vi "Get Video Image.vi"(8 "error in (no error)":errorcluster, 9 "Wait For Next Image?":bool=TRUE, 10 "Flip Image?":bool=TRUE, 11 "queue in":refnum<queue>) -> (0 "error out":errorcluster, 1 "Image Is New?":bool, 2 "Video Image Pixels (U32)":u32[][](array[numeric]), 3 "Video Image":T1(plugin-control))   [LabVIEW 2010, in "Kinect_API.lvlib"]
uses:
  Kinect_API.lvlib
  <vilib>/vision/Image Controls.llb/IMAQ Image.ctl
  <vilib>/vision/NI_Vision_Development_Module.lvlib
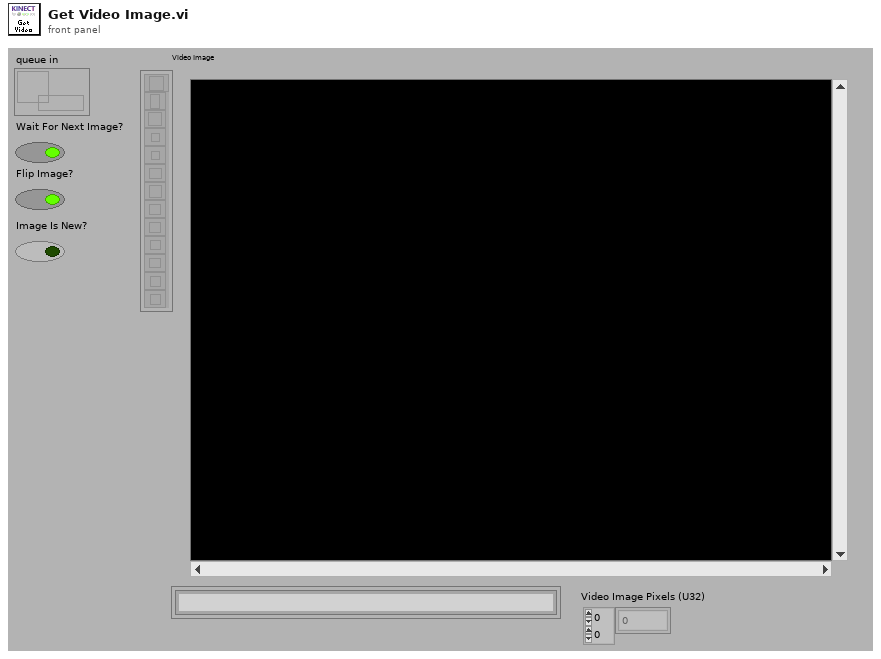
[diagram p1: front panel]
types:
  T1 = typedef "IMAQ Image.ctl" = refnum<image>
  T2 = typedef "Image Type" = u32
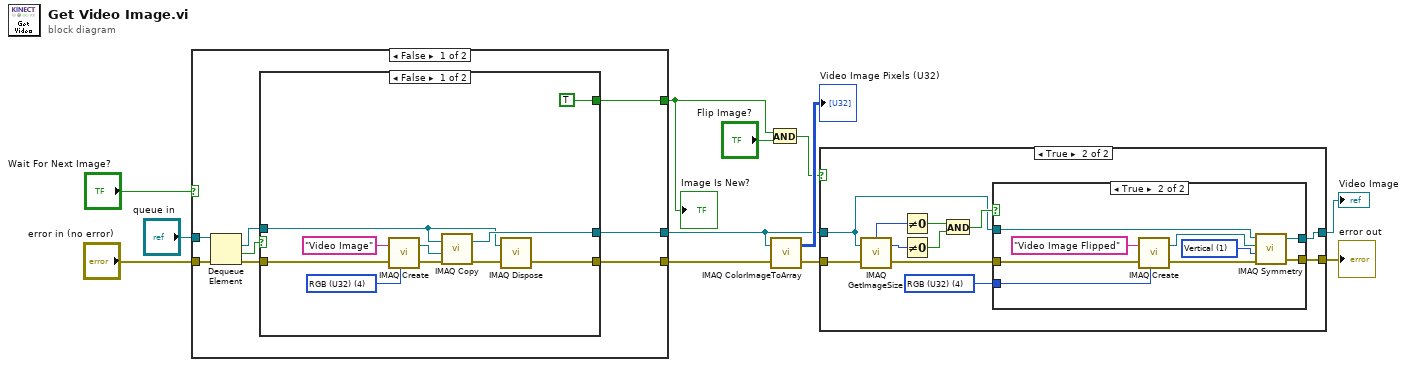
[diagram p0: block diagram]
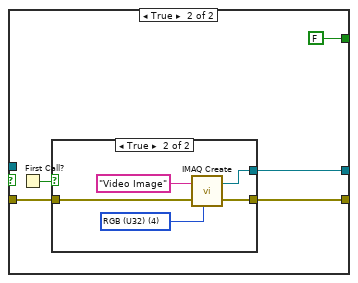
[diagram p4: hidden frame]
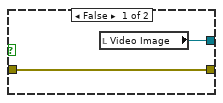
[diagram p5: hidden frame]
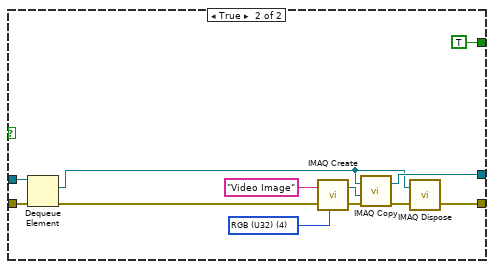
[diagram p6: hidden frame]
diagram:
  n1 = case shown="False" "Wait For Next Image?" {
    tunnel: "error in (no error)" -> [w16 w54]
    tunnel: [w18 w48] -> w7
    tunnel: [w19 w44] -> w8
    tunnel: [w20 TRUE] -> w2
    tunnel: "queue in" -> [w17 w52]
    frame False {
      n2 = Dequeue Element(queue=w17, error in (no error)=w16) -> (element=w13:T1, timed out?=w14:bool, error out=w15:errorcluster)  [unwired: 1 in, 1 out]
      n3 = case shown="False" w14 {
        tunnel: [w24 w31] -> w18
        tunnel: w15 -> [w21 w33]
        tunnel: [w23 w32] -> w19
        tunnel: [TRUE FALSE] -> w20
        tunnel: w13 -> [w22 _]
        frame False {
          w26 = T2 4 items=["Grayscale (U8)", "Grayscale (I16)", "Grayscale (SGL)", "Complex (CSG)", "RGB (U32)", "HSL (U32)", "RGB (U64)", "Grayscale (U16)"] ("Image Type")
          n4 = call "IMAQ Create"("Image Name"="Video Image", "Image Type"=w26, "error in (no error)"=w21) -> ("New Image"=w28:T1, "error out"=w27:errorcluster)  [unwired: 2 in]
          n5 = call "IMAQ Copy"("error in (no error)"=w27, "Image Dst"=w28, "Image Src"=w22) -> ("error out"=w25:errorcluster, "Image Dst Out"=w24:T1)  [unwired: 3 in]
          n6 = call "IMAQ Dispose"("Image"=w22, "error in (no error)"=w25) -> ("error out"=w23:errorcluster)  [unwired: 4 in]
        }
        frame True {
          n7 = First Call?() -> (First Call?: T/F=w34:bool)
          n8 = case shown="True" w34 {
            tunnel: [w37 w38] -> w31
            tunnel: w33 -> [w36 w40]
            tunnel: [w36 w39] -> w32
            frame False {
              n9 = local read "Video Image"() -> (w37:T1)
            }
            frame True {
              w41 = T2 4 items=["Grayscale (U8)", "Grayscale (I16)", "Grayscale (SGL)", "Complex (CSG)", "RGB (U32)", "HSL (U32)", "RGB (U64)", "Grayscale (U16)"] ("Image Type")
              n10 = call "IMAQ Create"("Image Name"="Video Image", "Image Type"=w41, "error in (no error)"=w40) -> ("New Image"=w38:T1, "error out"=w39:errorcluster)  [unwired: 2 in]
            }
          }
        }
      }
    }
    frame True {
      w46 = T2 4 items=["Grayscale (U8)", "Grayscale (I16)", "Grayscale (SGL)", "Complex (CSG)", "RGB (U32)", "HSL (U32)", "RGB (U64)", "Grayscale (U16)"] ("Image Type")
      n11 = Dequeue Element(queue=w52, error in (no error)=w54) -> (element=w43:T1, error out=w50:errorcluster)  [unwired: 1 in, 2 out]
      n12 = call "IMAQ Create"("Image Name"="Video Image", "Image Type"=w46, "error in (no error)"=w50) -> ("New Image"=w49:T1, "error out"=w47:errorcluster)  [unwired: 2 in]
      n13 = call "IMAQ Copy"("error in (no error)"=w47, "Image Dst"=w49, "Image Src"=w43) -> ("error out"=w45:errorcluster, "Image Dst Out"=w48:T1)  [unwired: 3 in]
      n14 = call "IMAQ Dispose"("Image"=w43, "error in (no error)"=w45) -> ("error out"=w44:errorcluster)  [unwired: 4 in]
    }
  }
  "Image Is New?" <- w2
  n15 = And(x=w2, y="Flip Image?") -> (x .and. y?=w1:bool)
  n16 = call "IMAQ ColorImageToArray"("Image"=w7, "error in (no error)"=w8) -> ("Image Pixels (U32)"=→"Video Image Pixels (U32)":u32[][], "error out"=w6:errorcluster)  [unwired: 2 in, 1 out]
  n17 = case shown="True" w1 {
    tunnel: w7 -> [w56 w57]
    tunnel: [w56 w67] -> w4
    tunnel: w6 -> [w55 w62]
    tunnel: [w55 w66] -> w5
    frame False {
    }
    frame True {
      w65 = T2 4 items=["Grayscale (U8)", "Grayscale (I16)", "Grayscale (SGL)", "Complex (CSG)", "RGB (U32)", "HSL (U32)", "RGB (U64)", "Grayscale (U16)"] ("Image Type")
      n18 = call "IMAQ GetImageSize"("Image"=w57, "error in (no error)"=w62) -> ("Y Resolution"=w64:i32, "X Resolution"=w63:i32, "error out"=w61:errorcluster)  [unwired: 2 in]
      n19 = Not Equal To 0?(x=w63) -> (x != 0?=w60:bool)
      n20 = Not Equal To 0?(x=w64) -> (x != 0?=w59:bool)
      n21 = And(x=w60, y=w59) -> (x .and. y?=w58:bool)
      n22 = case shown="True" w58 {
        tunnel: [w69 w77] -> w67
        tunnel: [w68 w76] -> w66
        tunnel: w65 -> [_ w75]
        tunnel: w61 -> [w68 w72]
        tunnel: w57 -> [w69 w71]
        frame False {
        }
        frame True {
          w78 = u32 1 items=["Horizontal", "Vertical", "Central", "1st Diagonal", "2nd Diagonal"] ("Type of Symmetry")
          n23 = call "IMAQ Create"("Image Name"="Video Image Flipped", "Image Type"=w75, "error in (no error)"=w72) -> ("New Image"=w74:T1, "error out"=w73:errorcluster)  [unwired: 2 in]
          n24 = call "IMAQ Symmetry"("error in (no error)"=w73, "Type of Symmetry"=w78, "Image Dst"=w74, "Image Src"=w71) -> ("error out"=w76:errorcluster, "Image Dst Out"=w77:T1)  [unwired: 1 in]
        }
      }
    }
  }
  "Video Image" <- w4
  "error out" <- w5
